vi "New Log File Configuration.vi"(8 "error in (no error)":errorcluster, 9 "Default Log File Path":string[](array[string]), 10 "Default Section Name":string="Log File", 11 "Device Ref in":T1=18446744073709551615 format="%.0x") -> (0 "error out":errorcluster, 3 "Device Ref out":T1 format="%.0x")   [LabVIEW 2019, in "Telemetry System Explorer.lvlib"]
uses:
  Telemetry System Explorer.lvlib
  <vilib>/NI VeriStand/Custom Device API/Custom Device Item Ref.ctl
  Shared/Constants.vi
  <vilib>/NI VeriStand/Custom Device API/Set Item Property (String Array).vi
  <vilib>/NI VeriStand/Custom Device API/Set Item Property (Boolean).vi
  <vilib>/NI VeriStand/Custom Device API/Custom Device API.lvlib
  Shared/Telemetry Shared.lvlib
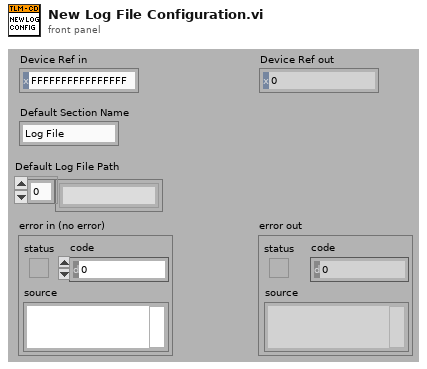
[diagram p1: front panel]
types:
  T1 = typedef "Custom Device API.lvlib/Custom Device Item Ref.ctl" = u64
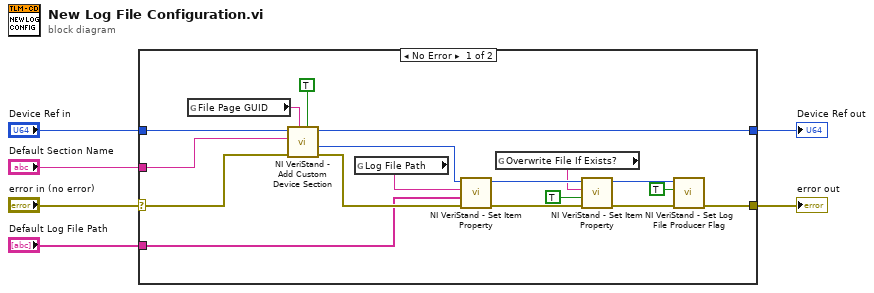
[diagram p0: block diagram]
diagram:
  n1 = case shown="No Error" "error in (no error)" {
    selector: "error in (no error)" -> [w15 w25]
    tunnel: "Default Section Name" -> [w23 _]
    tunnel: "Default Log File Path" -> [w10 _]
    tunnel: "Device Ref in" -> [w17 w26]
    tunnel: [w16 w26] -> w3
    tunnel: [w11 w25] -> w2
    frame No Error {
      n2 = global read "Constants.vi" "File Page GUID"() -> (w9:string)
      n3 = call <vilib>:"NI VeriStand - Add Custom Device Section.vi"("Highlight? (F)"=TRUE, "GUID (Default Section)"=w9, "error in (no error)"=w15, "Section Name"=w23, "Parent Ref in"=w17) -> ("error out"=w24:errorcluster, "Section Ptr"=w18:T1, "Parent Ref out"=w16:T1)  [unwired: 2 in, 2 out]
      n4 = global read "Constants.vi" "Log File Path"() -> (w8:string)
      n5 = call-poly <vilib>:"NI VeriStand - Set Item Property.vi"("error in (no error)"=w24, "Value"=w10, "Property Name"=w8, "Item Ref in"=w18) -> ("error out"=w21:errorcluster, "Item Ref out"=w22:T1)  [unwired: 6 out]
      n6 = global read "Constants.vi" "Overwrite File If Exists?"() -> (w7:string)
      n7 = call-poly <vilib>:"NI VeriStand - Set Item Property.vi"("error in (no error)"=w21, "Value"=TRUE, "Property Name"=w7, "Item Ref in"=w22) -> ("error out"=w13:errorcluster, "Item Ref out"=w14:T1)  [unwired: 6 out]
      n8 = call <vilib>:"NI VeriStand - Set Log File Producer Flag.vi"("error in (no error)"=w13, "Log File Producer"=TRUE ("Log File Provider"), "Item Ref in"=w14) -> ("error out"=w11:errorcluster)  [unwired: 7 in, 1 out]
    }
    frame Error {
    }
  }
  "Device Ref out" <- w3
  "error out" <- w2
